vi "Debug Command.vi"(0 "BoardHandle":T1, 1 "No Channel":bool, 2 "Channel (0)":u8, 3 "All Channels (F)":bool, 5 "CMD":u8(ring) items=["MON", "SET", "INFO"], 7 "PAR":string(combo)="BDNAME", 9 "VAL":string, 11 "error in (no error)":errorcluster) -> (4 "BoardHandle out":T1, 6 "Command":string, 8 "Response":string, 10 "val":string, 15 "error out":errorcluster)   [LabVIEW 2020, in "CAEN PSM.lvlib"]
doc: "This function can be used for debug purpose. This allows to prepare and forward a command and view the received response string."
uses:
  CAEN PSM.lvlib
  Private/BoardHandle.ctl
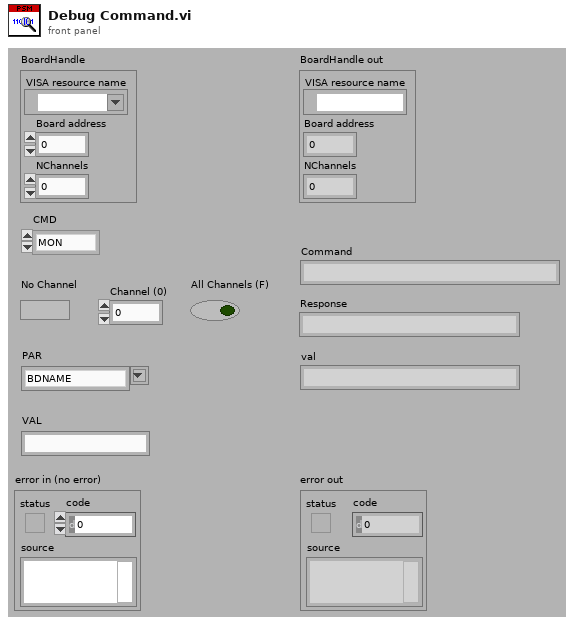
[diagram p1: front panel]
types:
  T1 = typedef "CAEN PSM.lvlib/BoardHandle.ctl" = cluster{"VISA resource name":refnum<visa-resource-name>, "Board address":i8, "NChannels":u8}
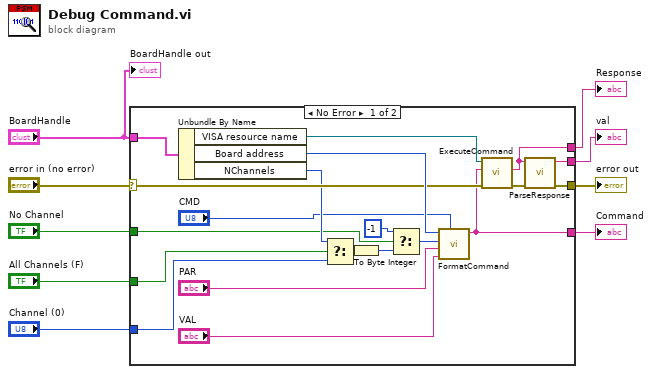
[diagram p0: block diagram]
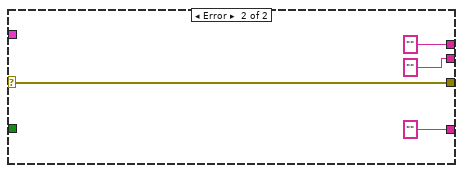
[diagram p2: hidden frame]
diagram:
  n1 = case shown="No Error" "error in (no error)" {
    selector: "error in (no error)" -> [w24 w33]
    tunnel: "All Channels (F)" -> [w22 _]
    tunnel: "Channel (0)" -> [w28 _]
    tunnel: [w21 w33] -> w6
    tunnel: "BoardHandle" -> [w25 _]
    tunnel: [w20 "" ("val")] -> w4
    tunnel: [w19 "" ("Response")] -> w3
    tunnel: [w18 "" ("cmd")] -> w2
    tunnel: "No Channel" -> [w14 _]
    frame No Error {
      n2 = Unbundle By Name(w25) -> ("VISA resource name"=w27:refnum<visa-resource-name>, "Board address"=w29:i8, "NChannels"=w23:u8)
      n3 = Select(t=w23, s=w22, f=w28) -> (s? t:f=w12:u8)
      n4 = To Byte Integer(number=w12) -> (8bit integer=w10:i8)
      n5 = Select(t=i8 -1, s=w14, f=w10) -> (s? t:f=w11:i8)
      n6 = call "FormatCommand.vi"("CMD (MON)"="CMD", "VAL"="VAL", "PAR"="PAR", "CH"=w11, "BD (0)"=w29) -> ("cmd"=w18:string)  [unwired: 6 in]
      n7 = call "ExecuteCommand.vi"("error in (no error)"=w24, "Command"=w18, "VISA resource name"=w27) -> ("error out"=w26:errorcluster, "Response"=w19:string)  [unwired: 6 in, 1 out]
      n8 = call "ParseResponse.vi"("error in (no error)"=w26, "Response"=w19) -> ("error out"=w21:errorcluster, "val"=w20:string)  [unwired: 6 in, 2 out]
    }
    frame Error {
    }
  }
  "error out" <- w6
  "val" <- w4
  "Response" <- w3
  "Command" <- w2
  "BoardHandle out" <- "BoardHandle"
